vi "Reading the file improved.vi"() -> ()   [LabVIEW 2020]
uses:
  Tools/Reflector/RFH-Reflection_File_Handler.lvlib
panel:
  out "string array 4":string[](array[string])
  out "string array 3":string[](array[string])
  out "deleted portion":string[](array[string])
  out "Numeric":i32
  out "substring":string
  out "trimmed string":string
  out "string array 2":string[](array[string])
  out "string array":string[](array[string])
  out "offset past match":i32
  out "after substring":string
  out "match substring":string
  out "before substring":string
  in  "error in":errorcluster
  in  "file path (dialog if empty)":path
  out "text":string
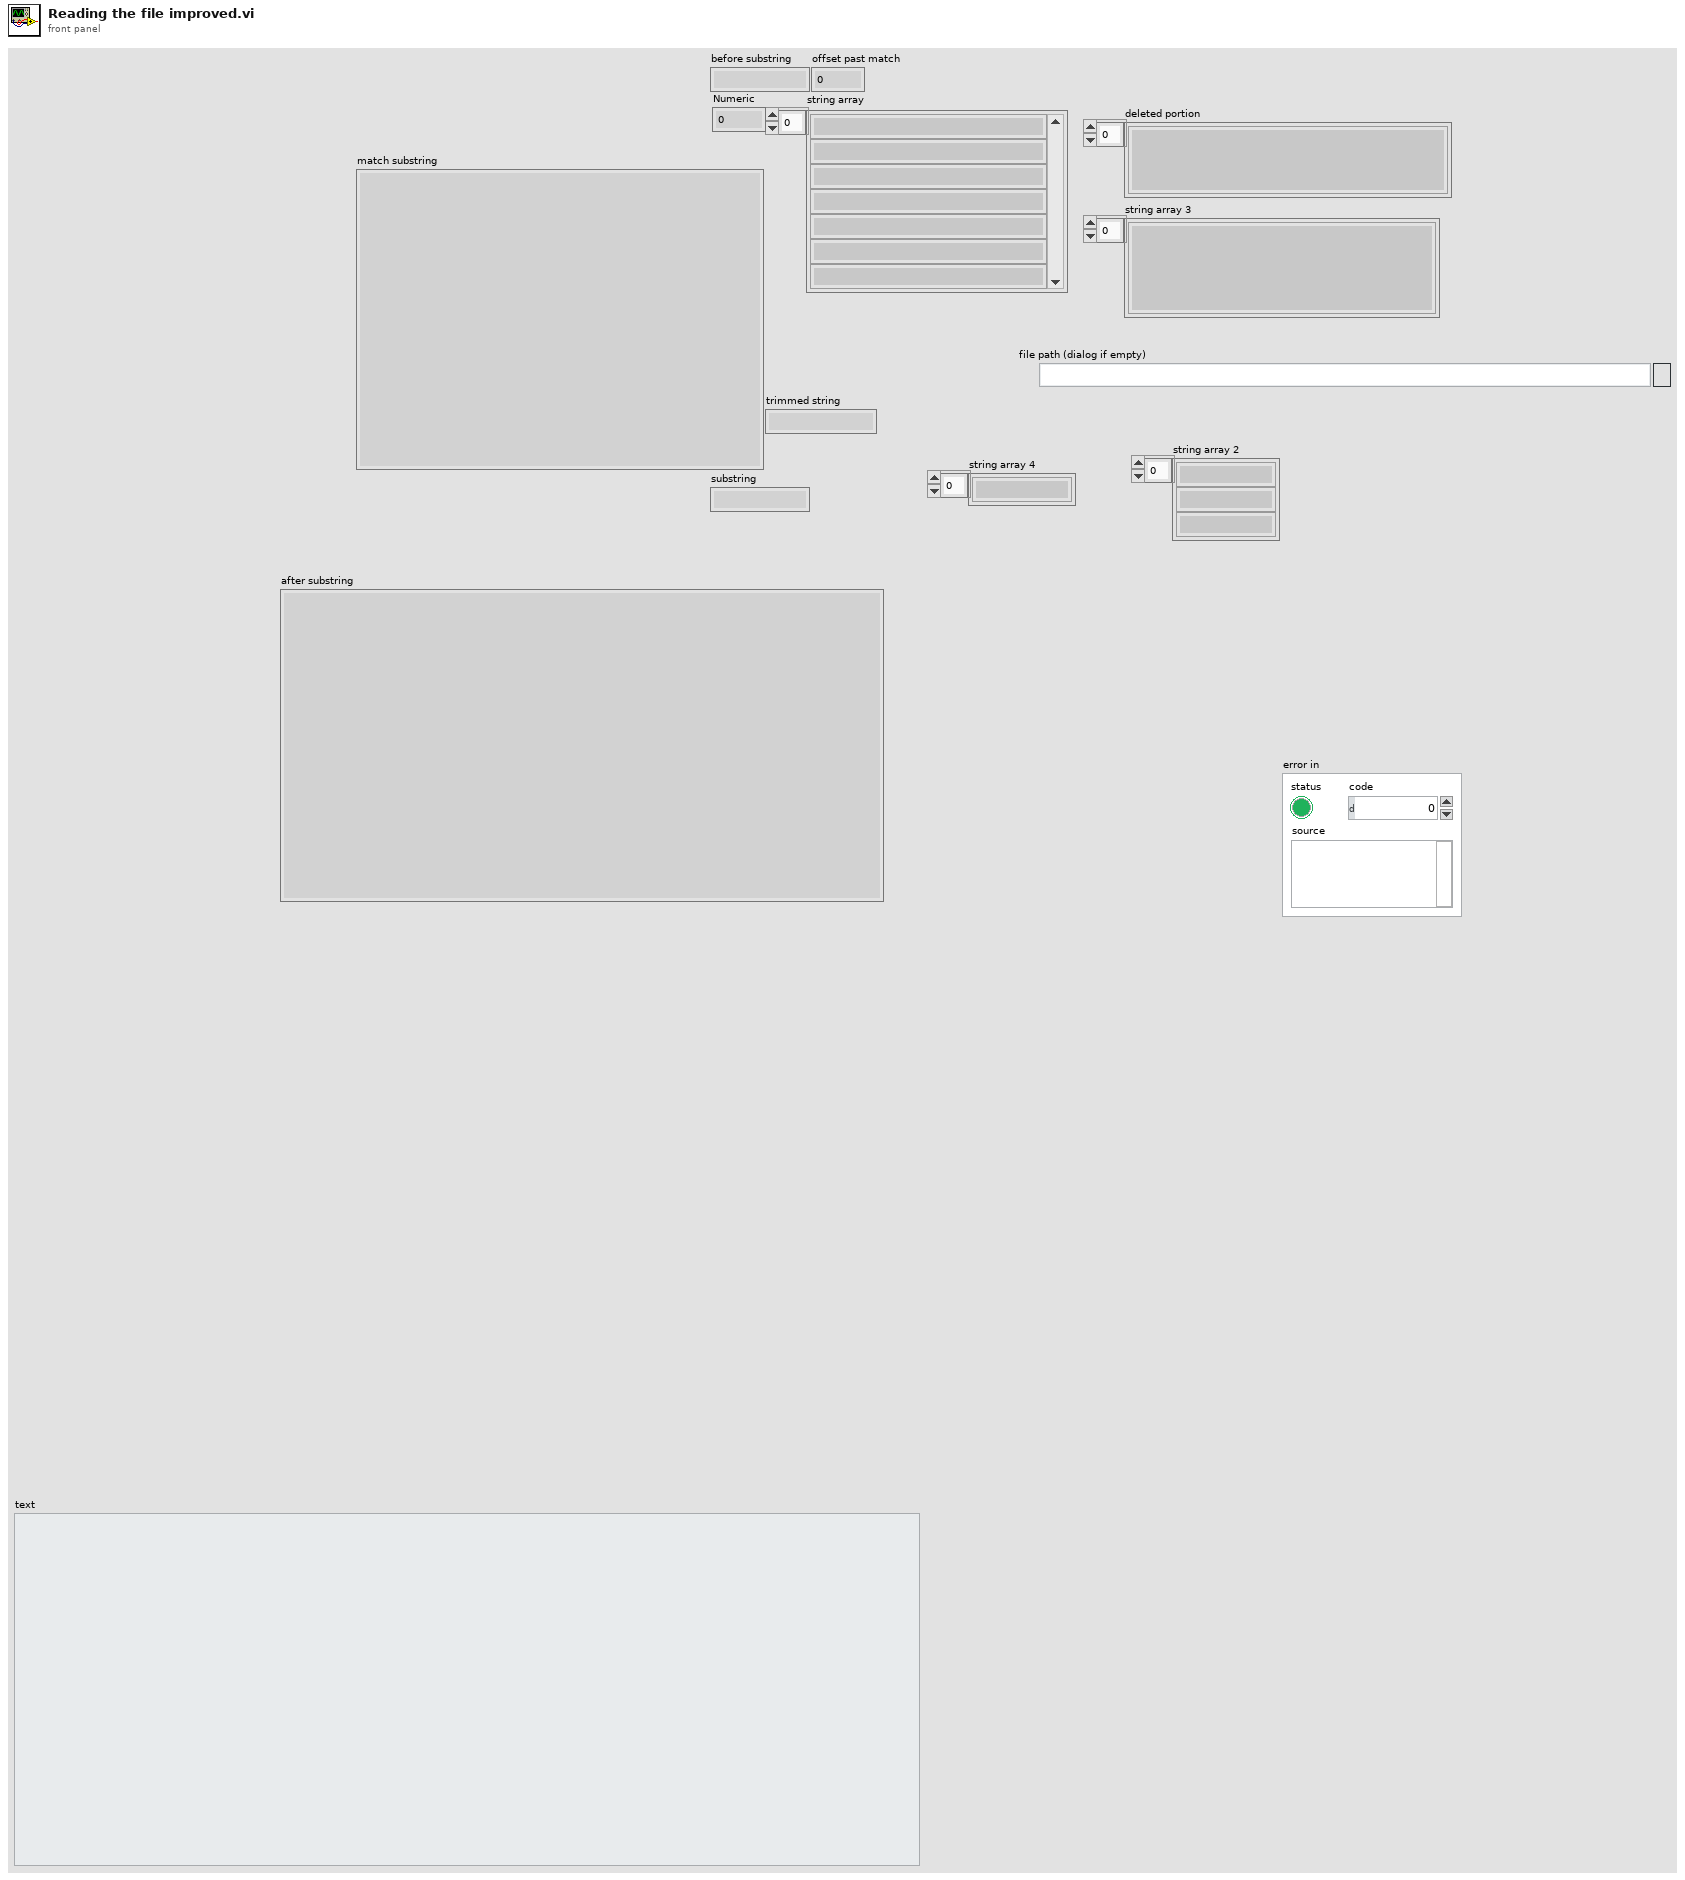
[diagram p1: front panel]
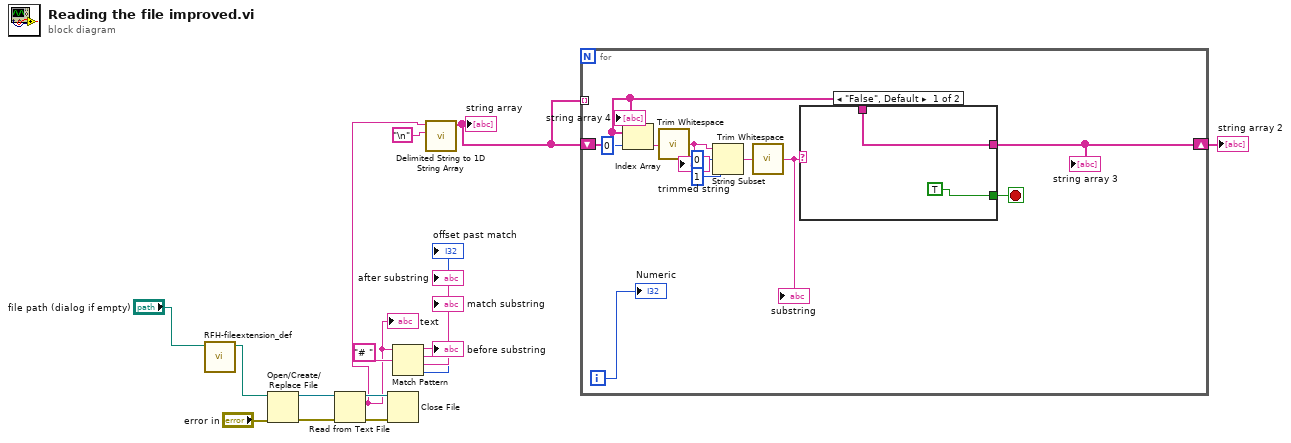
[diagram p0: block diagram]
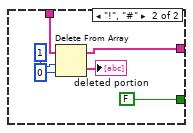
[diagram p2: hidden frame]
diagram:
  n1 = call "RFH-fileextension_def.vi"("Path in"="file path (dialog if empty)") -> ("Path with file extention"=w9:path)  [unwired: 9 in, 1 out]
  n2 = Open/Create/Replace File(file path (use dialog)=w9, error in="error in") -> (refnum out=w16:refnum<file>, error out=w13:errorcluster)  [unwired: 4 in, 1 out]
  n3 = Read from Text File(file (use dialog)=w16, error in=w13) -> (refnum out=w15:refnum<file>, text=w3:string, error out=w14:errorcluster)  [unwired: 2 in, 1 out]
  "text" <- w3
  n4 = Close File(refnum=w15, error in=w14) -> ()  [unwired: 2 out]
  n5 = Match Pattern(string=w3, regular expression="# " ("search string/char (-)")) -> (before substring=→"before substring":string, match substring=→"match substring":string, after substring=→"after substring":string, offset past match=→"offset past match":i32)  [unwired: 1 in]
  n6 = call <vilib>:"Delimited String to 1D String Array.vi"("delimiter"="\n", "delimited string"=w3) -> ("string array"=w1:string[])  [unwired: 9 in]
  "string array" <- w1
  n7 = for {
    shift-right: [w20] -> w2
    shift-left: w1 -> [w21]
    tunnel: w1 -> [_] mode=indexing
    i -> [w23]
    stop <- w19 stop-if-true
    n8 = Index Array(array=w21, index=0) -> (element=w22:string)
    n9 = call <vilib>:"Trim Whitespace.vi"("string"=w22) -> ("trimmed string"=w27:string)  [unwired: 1 in]
    "trimmed string" <- w27
    n10 = String Subset(string=w27, offset (0)=0, length (rest)=1 ("length (rest)")) -> (substring=w24:string)
    n11 = call <vilib>:"Trim Whitespace.vi"("string"=w24) -> ("trimmed string"=w18:string)  [unwired: 1 in]
    "substring" <- w18
    n12 = case shown="\"False\", Default" w18 {
      tunnel: w21 -> [w29 w35]
      tunnel: [w29 w32] -> w20
      tunnel: [TRUE FALSE] -> w19
      frame "False", Default {
      }
      frame "!", "#" {
        n13 = Delete From Array(array=w35, length=1, index=0) -> (deleted portion=→"deleted portion":string[], array with subset deleted=w32:string[])
      }
    }
    "string array 3" <- w20
    "Numeric" <- w23
    "string array 4" <- w21
  }
  "string array 2" <- w2
